vi "myRIO_BRig_RT_dataBlock_targetTpB__R.vi"() -> (2 "output_targetTpB__R":i32)   [LabVIEW 2014]
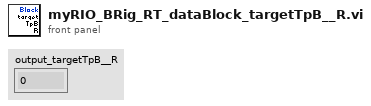
[diagram p1: front panel]
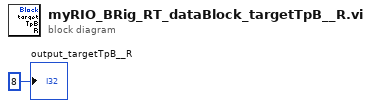
[diagram p0: block diagram]
diagram:
  "output_targetTpB__R" <- 8 ("output_iBlock")
